vi "TCS_Rx_VISA.vi"() -> ()   [LabVIEW 2018]
uses:
  RxTx/RxTx.lvclass
  Serial Communication/Serial Communication.lvclass
  Serial Communication/Serial Communication.lvclass/Serial Communication.ctl
panel:
  in  "Serial Communication in":refnum<class "Serial Communication.lvclass">
  in  "VISA resource name":refnum<visa-resource-name>
  in  "RxTx in":refnum<class "RxTx.lvclass">
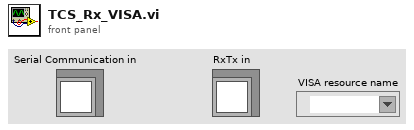
[diagram p1: front panel]
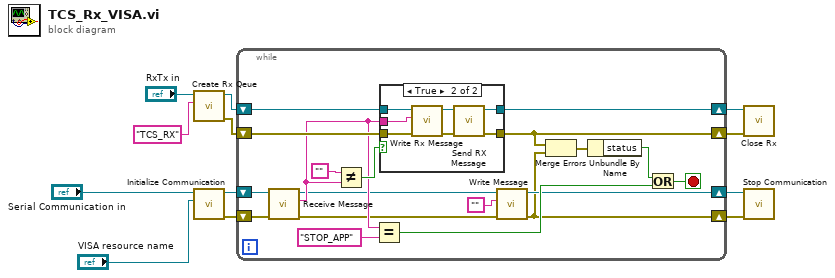
[diagram p0: block diagram]
diagram:
  n1 = call "Create Rx Qeue.vi"("Reader Name"="TCS_RX", "RxTx in"="RxTx in") -> ("error out"=w9:errorcluster, "RxTx out"=w10:refnum<class "RxTx.lvclass">)  [unwired: 8 in]
  n2 = call "Initialize Communication.vi"("VISA resource name"="VISA resource name", "Serial Communication in"="Serial Communication in") -> ("error out"=w5:errorcluster, "Serial Communication out"=w6:refnum<class "Serial Communication.lvclass">)  [unwired: 8 in]
  n3 = while {
    shift-right: [w16] -> w1
    shift-left: w5 -> [w19]
    shift-right: [w17] -> w2
    shift-left: w6 -> [w20]
    shift-right: [w21] -> w11
    shift-left: w9 -> [w31]
    shift-right: [w29] -> w12
    shift-left: w10 -> [w30]
    stop <- w24 stop-if-true
    n4 = call "Receive Message.vi"("error in (no error)"=w19, "Serial Communication in"=w20) -> ("error out"=w14:errorcluster, "Message"=w18:string, "Serial Communication out"=w15:refnum<class "Serial Communication.lvclass">)  [unwired: 7 in]
    n5 = Not Equal?(x="", y=w18) -> (x != y?=w26:bool)
    n6 = Equal?(x=w18, y="STOP_APP" ("reader name")) -> (x = y?=w22:bool)
    n7 = case shown="True" w26 {
      tunnel: w31 -> [w32 w36]
      tunnel: w30 -> [w33 w35]
      tunnel: [w33 w40] -> w29
      tunnel: [w32 w39] -> w21
      tunnel: w18 -> [_ w34]
      frame False {
      }
      frame True {
        n8 = call "Write Rx Message.vi"("error in (no error)"=w36, "Rx message"=w34, "RxTx in"=w35) -> ("error out"=w37:errorcluster, "RxTx out"=w38:refnum<class "RxTx.lvclass">)  [unwired: 7 in]
        n9 = call "Send RX Message.vi"("error in (no error)"=w37, "RxTx in"=w38) -> ("error out"=w39:errorcluster, "RxTx out"=w40:refnum<class "RxTx.lvclass">)  [unwired: 8 in]
      }
    }
    n10 = call "Write Message.vi"("error in (no error)"=w14, "Message"="", "Serial Communication in"=w15) -> ("error out"=w16:errorcluster, "Serial Communication out"=w17:refnum<class "Serial Communication.lvclass">)  [unwired: 7 in]
    n11 = Merge Errors(w21, w16) -> (w28:errorcluster)
    n12 = Unbundle By Name(w28) -> ("status"=w23:bool)
    n13 = Or(x=w23, y=w22) -> (x .or. y?=w24:bool)
  }
  n14 = call "Close Rx.vi"("error in (no error)"=w11, "RxTx in"=w12) -> ()  [unwired: 8 in, 2 out]
  n15 = call "Stop Communication.vi"("error in (no error)"=w1, "Serial Communication in"=w2) -> ()  [unwired: 8 in, 2 out]
